vi "3C SetpointsToTCP.vi"(10 "remote port or service name":u16=10001, 11 "address":string="192.168.1.11") -> (0 "error out":errorcluster, 3 "TCP Connected?":bool)   [LabVIEW 2011]
uses:
  2-Think/2 Typedefs/setpoints to boat.ctl
  2-Think/2 Typedefs/sail setpt.ctl
  2-Think/2 Typedefs/rudder angle.ctl
  2-Think/2 Typedefs/generalized actuator status.ctl
  2-Think/2 Typedefs/indicator LED.ctl
  2-Think/2 Globals/2 Global.vi
panel:
  out "Output Array":u8[](array[numeric])
  out "Setpoints to boat out":T1
  in  "VI Stop":bool
  # "This is the Set-Points to TCP writer.\n\nThis vi reads the global variable setpoints and passes them through to the TCP connection.\n\nTODO: make it actually work. Connection to the global variable seems a bit glitchy, as does the TCP connection."
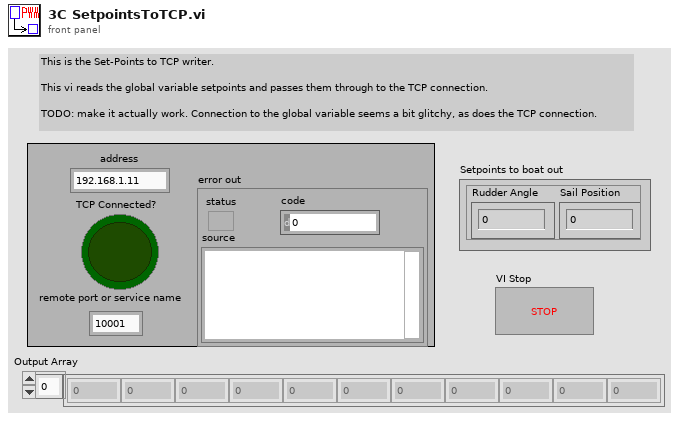
[diagram p1: front panel]
types:
  T1 = typedef "setpoints to boat.ctl" = cluster{"Sail Position":T2, "Rudder Angle":T3}
  T2 = typedef "sail setpt.ctl" = dbl
  T3 = typedef "rudder angle.ctl" = dbl
  T4 = typedef "generalized actuator status.ctl" = cluster{"Actuator Connected":T5}
  T5 = typedef "indicator LED.ctl" = bool
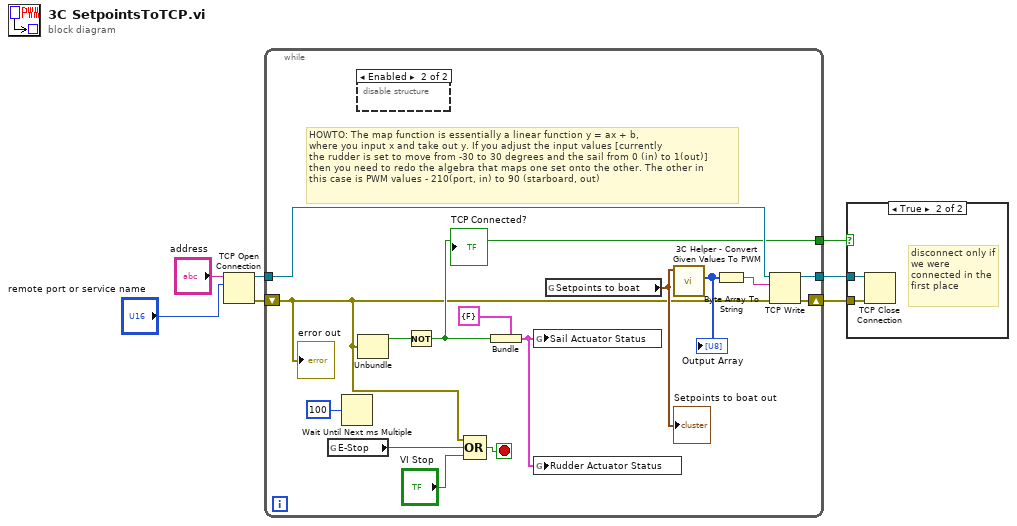
[diagram p0: block diagram]
diagram:
  n1 = TCP Open Connection(address="address", remote port or service name="remote port or service name") -> (connection ID=w4:refnum<k5>, error out=w5:errorcluster)  [unwired: 3 in]
  n2 = while {
    tunnel: w4 -> [w22]
    tunnel: [w21] -> w3
    tunnel: [w13] -> w2
    shift-right: [w12] -> w1
    shift-left: w5 -> [w8]
    stop <- w11 stop-if-true
    # "HOWTO: The map function is essentially a linear function y = ax + b,\nwhere you input x and take out y. If you adjust the input values [currently\nthe rudder is set to move from -30 to 30 degrees and the sail from 0 (in) to 1(out)]\nthen you need to redo the algebra that maps one set onto the other. The other in\nthis case is PWM values - 210(port, in) to 90 (starboard, out)"
    n3 = global read "2 Global.vi" "E-Stop"() -> (w9:bool)
    n4 = Wait Until Next ms Multiple(millisecond multiple=u32 100) -> ()  [unwired: 1 out]
    n5 = disable-structure shown="Enabled" {
      frame Disabled {
      }
      frame Enabled {
      }
    }
    n6 = Unbundle(w8) -> ("status"=w20:bool)  [unwired: 2 out]
    n7 = Not(x=w20) -> (.not. x?=w13:bool)
    "TCP Connected?" <- w13
    n8 = Compound Arithmetic op=OR(w8, w9, "VI Stop") -> (w11:bool)
    n9 = Bundle(cluster=T4 {"Actuator Connected"=FALSE} ("Sail Actuator Status"), "Actuator Connected"=w13) -> (w16:T4)
    n10 = global write "2 Global.vi" "Sail Actuator Status"(w16) -> ()
    n11 = global write "2 Global.vi" "Rudder Actuator Status"(w16) -> ()
    n12 = global read "2 Global.vi" "Setpoints to boat"() -> (w14:T1)
    "Setpoints to boat out" <- w14
    n13 = call "3C Helper - Convert Given Values To PWM.vi"("Setpoints to boat"=w14) -> ("Output Array, integers"=w15:u8[])  [unwired: 9 in, 1 out]
    "Output Array" <- w15
    n14 = Byte Array To String(unsigned byte array=w15) -> (string=w19:string)
    n15 = TCP Write(connection ID=w22, data in=w19, error in (no error)=w8) -> (connection ID out=w21:refnum<k5>, error out=w12:errorcluster)  [unwired: 1 in, 1 out]
    "error out" <- w8
  }
  n16 = case shown="True" w2 {
    tunnel: w1 -> [_ w24]
    tunnel: w3 -> [_ w23]
    frame False {
    }
    frame True {
      # "disconnect only if we were connected in the first place"
      n17 = TCP Close Connection(connection ID=w23, error in (no error)=w24) -> ()  [unwired: 1 in, 2 out]
    }
  }
